vi "XY Plot - Y Scale - Name Label Position Top--Const.vi"() -> (3 "Y Scale.Name Label.Position:Top":i32)   [LabVIEW 2017, in "DTacq Plot Display Library.lvlib"]
uses:
  DTacq Plot Display Library.lvlib
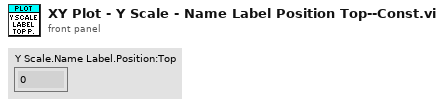
[diagram p1: front panel]
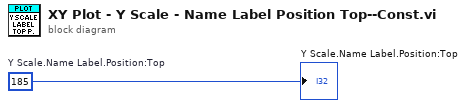
[diagram p0: block diagram]
diagram:
  w1 = 185  # Y Scale.Name Label.Position:Top
  "Y Scale.Name Label.Position:Top" <- w1
